vi "Next Step.vi"(8 "error in (no error)":errorcluster, 11 "Analog Out Scan in":refnum<class "Analog Output Scan.lvclass">) -> (0 "error out":errorcluster, 1 "Current Step":u32, 2 "Current Position":dbl, 3 "Analog Out Scan out":refnum<class "Analog Output Scan.lvclass">)   [LabVIEW 2017, in "Analog Output Scan.lvclass"]
doc: "(Dynamic) Move to the next preconfigured step of this Scanner, and return the current position (actual, not intended) of this Scanner. Increment the step counter by one."
uses:
  Analog Output Scan.lvclass
  Analog Output Scan.lvclass/Analog Output Scan.ctl
  <vilib>/DAQmx/write.llb/DAQmx Write (Analog DBL 1Chan 1Samp).vi
  <vilib>/DAQmx/miscellaneous.llb/DAQmx Fill In Error Info.vi
  Scanner/Scanner.lvclass
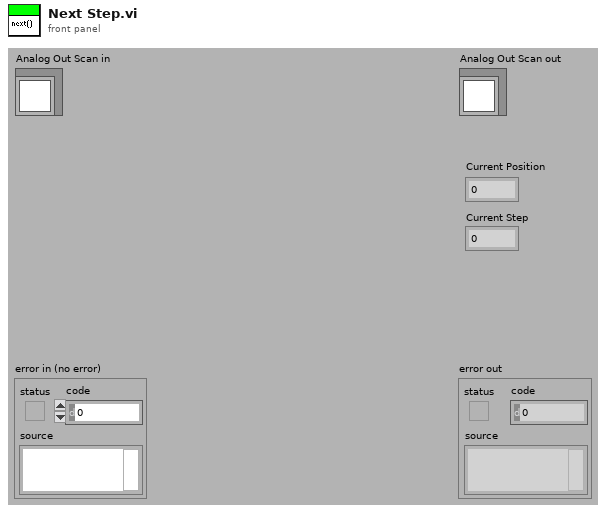
[diagram p1: front panel]
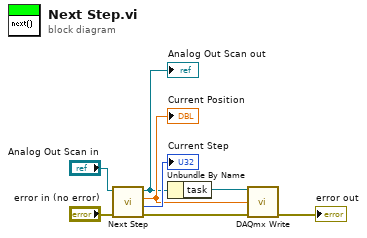
[diagram p0: block diagram]
diagram:
  n1 = call-parent "Next Step.vi"("error in (no error)"="error in (no error)", "Scanner in"="Analog Out Scan in") -> ("error out"=w3:errorcluster, "Current Step"=→"Current Step":u32, "Current Position"=w4:dbl, "Scanner out"=w2:refnum<class "Analog Output Scan.lvclass">)  [unwired: 6 in]
  "Analog Out Scan out" <- w2
  "Current Position" <- w4
  n2 = Unbundle By Name(w2) -> ("task"=w1:refnum<k21>)
  n3 = call-poly <vilib>:"DAQmx Write.vi"("task/channels in"=w1, "data"=w4, "error in"=w3) -> ("error out"=→"error out":errorcluster)  [unwired: 10 in, 2 out]
